vi "File.MD5Checksum Files.vi"(8 "error in (no error)":errorcluster, 11 "FilePaths":path[](array[path])) -> (0 "error out":errorcluster, 3 "MD5 message-digest":string)   [LabVIEW 2010]
doc: "Create an MD5 message-digest for a list of files."
uses:
  <userlib>/_OpenG.lib/md5/md5.llb/MD5 Message Digest (Hexadecimal String)__ogtk.vi
panel:
  out "MD5 Array":string[](array[string])
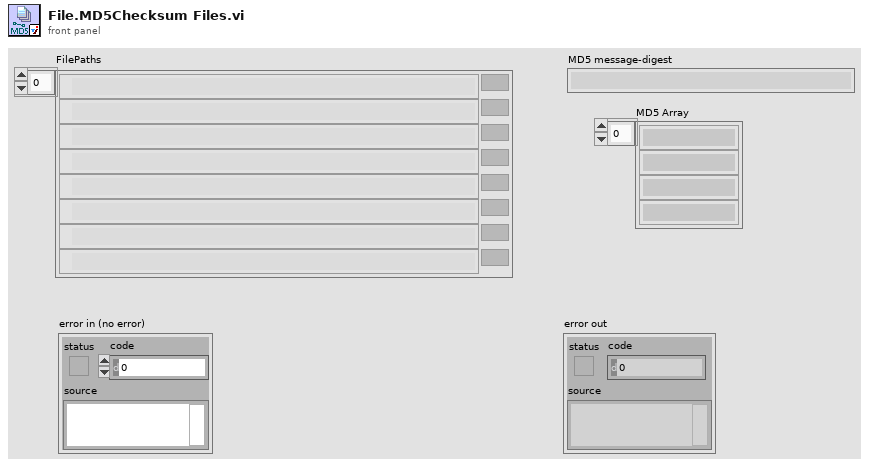
[diagram p1: front panel]
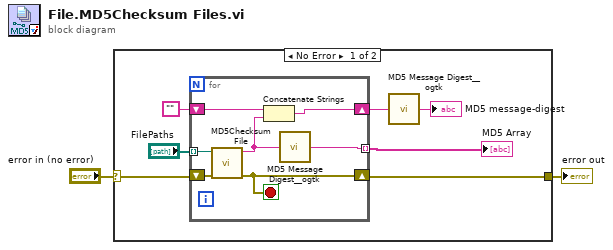
[diagram p0: block diagram]
diagram:
  n1 = case shown="No Error" "error in (no error)" {
    selector: "error in (no error)" -> [w5 w17]
    tunnel: [w8 w17] -> w1
    frame No Error {
      n2 = for {
        shift-right: [w12] -> w8
        shift-left: w5 -> [w15]
        tunnel: "FilePaths" -> [w16] mode=indexing
        shift-right: [w13] -> w7
        shift-left: "" -> [w14]
        tunnel: [w10] -> w3 mode=indexing
        stop <- w12 stop-if-true
        n3 = call <vilib>:"MD5Checksum File.vi"("error in (no error)"=w15, "Path"=w16) -> ("error out"=w12:errorcluster, "MD5 message-digest"=w11:string)  [unwired: 8 in]
        n4 = Concatenate Strings(w14, w11) -> (w13:string)
        n5 = call-poly <userlib>:"MD5 Message Digest__ogtk.vi"("Message"=w11) -> ("MD5 Message Digest"=w10:string)
      }
      "MD5 Array" <- w3
      n6 = call-poly <userlib>:"MD5 Message Digest__ogtk.vi"("Message"=w7) -> ("MD5 Message Digest"=→"MD5 message-digest":string)
    }
    frame Error {
    }
  }
  "error out" <- w1
